vi "FTW-dotNET-MySQL-CloseConnection.vi"(0 "DB Connection":refnum<k24>, 11 "error in":errorcluster) -> (15 "error out":errorcluster)   [LabVIEW 2015]
uses:
  C:/Program Files (x86)/MySQL/MySQL Installer for Windows/MySql.Data.dll
  Program Files (x86)/MySQL/MySQL Installer for Windows/MySql.Data.dll
panel:
  # "Inputs"
  # "Outputs"
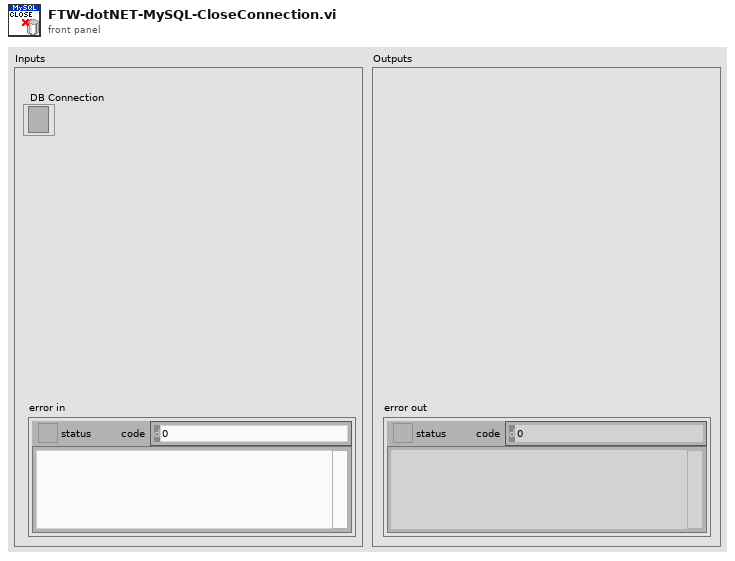
[diagram p1: front panel]
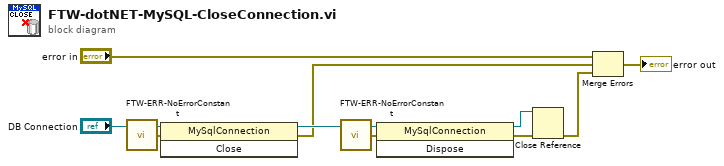
[diagram p0: block diagram]
diagram:
  n1 = call "FTW-ERR-NoErrorConstant.vi"() -> ("no error"=w9:errorcluster)
  n2 = invoke class="MySqlConnection" method="Close"(reference="DB Connection", error in=w9) -> (reference out=w7:refnum<k24>, error out=w6:errorcluster)  [unwired: 1 in, 1 out]
  n3 = call "FTW-ERR-NoErrorConstant.vi"() -> ("no error"=w8:errorcluster)
  n4 = invoke class="MySqlConnection" method="Dispose"(reference=w7, error in=w8) -> (reference out=w4:refnum<k24>, error out=w5:errorcluster)  [unwired: 1 in, 1 out]
  n5 = Close Reference(reference=w4, error in (no error)=w5) -> (error out=w3:errorcluster)
  n6 = Merge Errors("error in", w6, w3) -> (→"error out":errorcluster)
